vi "Auto Arms Down V.3.0.vi"() -> (3 "Stop":bool=TRUE)   [LabVIEW 2017]
uses:
  Robot Global Data V.3.0.vi
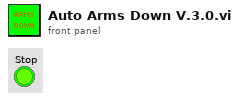
[diagram p1: front panel]
types:
  T1 = cluster{"Pot. Voltage":dbl[], "Corresponding Inches":dbl[]}
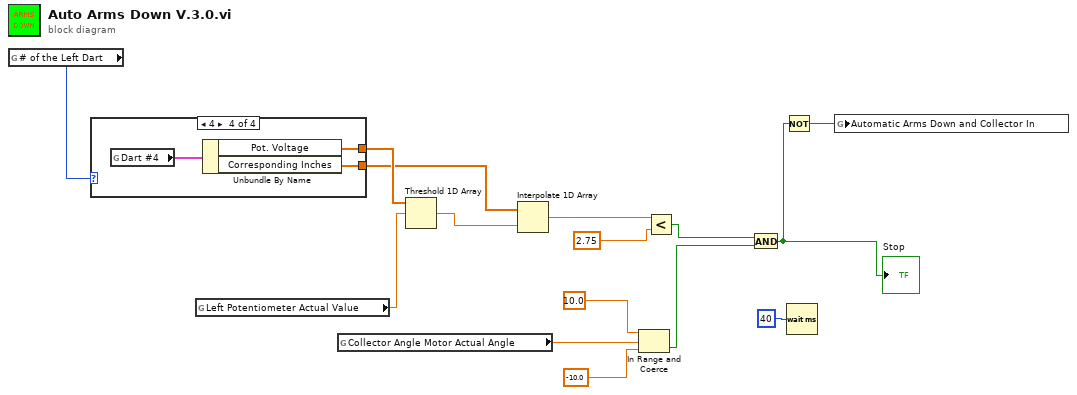
[diagram p0: block diagram]
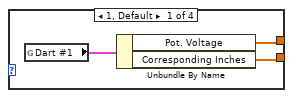
[diagram p2: hidden frame]
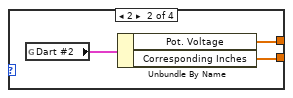
[diagram p3: hidden frame]
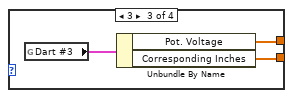
[diagram p4: hidden frame]
diagram:
  n1 = global read "Robot Global Data V.3.0.vi" "# of the Left Dart"() -> (w4:i32)
  n2 = case shown="4" w4 {
    tunnel: [w17 w20 w23 w26] -> w6
    tunnel: [w16 w19 w22 w25] -> w5
    frame 1, Default {
      n3 = global read "Robot Global Data V.3.0.vi" "Dart #1"() -> (w18:T1)
      n4 = Unbundle By Name(w18) -> ("Pot. Voltage"=w17:dbl[], "Corresponding Inches"=w16:dbl[])
    }
    frame 2 {
      n5 = global read "Robot Global Data V.3.0.vi" "Dart #2"() -> (w21:T1)
      n6 = Unbundle By Name(w21) -> ("Pot. Voltage"=w20:dbl[], "Corresponding Inches"=w19:dbl[])
    }
    frame 3 {
      n7 = global read "Robot Global Data V.3.0.vi" "Dart #3"() -> (w24:T1)
      n8 = Unbundle By Name(w24) -> ("Pot. Voltage"=w23:dbl[], "Corresponding Inches"=w22:dbl[])
    }
    frame 4 {
      n9 = global read "Robot Global Data V.3.0.vi" "Dart #4"() -> (w27:T1)
      n10 = Unbundle By Name(w27) -> ("Pot. Voltage"=w26:dbl[], "Corresponding Inches"=w25:dbl[])
    }
  }
  n11 = global read "Robot Global Data V.3.0.vi" "Left Potentiometer Actual Value"() -> (w7:dbl)
  n12 = global read "Robot Global Data V.3.0.vi" "Collector Angle Motor Actual Angle"() -> (w13:dbl)
  n13 = Threshold 1D Array(2:w7, 3:w6) -> (0:w8:dbl)  [unwired: 1 in]
  n14 = Interpolate 1D Array(1:w8, 2:w5) -> (0:w3:dbl)
  n15 = In Range and Coerce(upper limit=10.0, x=w13, lower limit=-10.0) -> (In Range?=w10:bool)  [unwired: 1 out]
  n16 = Less?(x=w3, y=2.75) -> (x < y?=w14:bool)
  n17 = And(x=w14, y=w10) -> (x .and. y?=w2:bool)
  "Stop" <- w2
  n18 = Not(x=w2) -> (.not. x?=w1:bool)
  n19 = Wait (ms)(milliseconds to wait=u32 40) -> ()  [unwired: 1 out]
  n20 = global write "Robot Global Data V.3.0.vi" "Automatic Arms Down and Collector In"(w1) -> ()
